vi "Untitled 1 (SubVI).vi"(11 "String":string) -> (3 "Array":dbl[](array[numeric]))   [LabVIEW 2018]
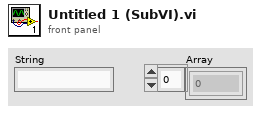
[diagram p1: front panel]
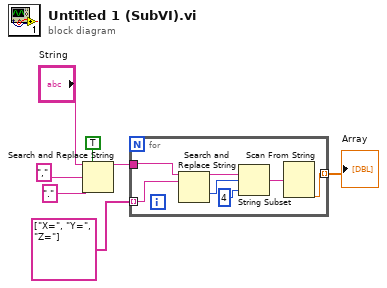
[diagram p0: block diagram]
diagram:
  n1 = Search and Replace String(replace all?=TRUE ("replace all? (F)"), input string="String", search string=".", replace string="," ("replace string (\"\")")) -> (result string=w1:string)  [unwired: 4 in, 3 out]
  n2 = for {
    tunnel: w1 -> [w14]
    tunnel: [w13] -> w7 mode=indexing
    tunnel: string[] ["X=", "Y=", "Z="] -> [w8] mode=indexing
    n3 = Search and Replace String(input string=w14, search string=w8) -> (result string=w12:string, offset past replacement=w11:i32)  [unwired: 6 in, 2 out]
    n4 = String Subset(string=w12, offset (0)=w11, length (rest)=4) -> (substring=w10:string)
    n5 = Scan From String(input string=w10) -> (output 1=w13:dbl)  [unwired: 4 in, 3 out]
  }
  "Array" <- w7
